vi "core_process_api_vi_ref.vi"(6 "pre/post":enum16{"pre", "post"}(ring), 8 "error in":errorcluster, 9 "vi path":path, 10 "name of caller in":string, 11 "api vi ref in":T1) -> (0 "error out":errorcluster, 3 "api vi ref out":T1)   [LabVIEW 2015]
uses:
  api_vi_ref.ctl
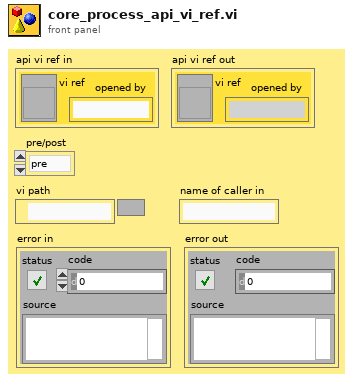
[diagram p1: front panel]
types:
  T1 = typedef "api_vi_ref.ctl" = cluster{"vi ref":refnum<vi>, "opened by":string}
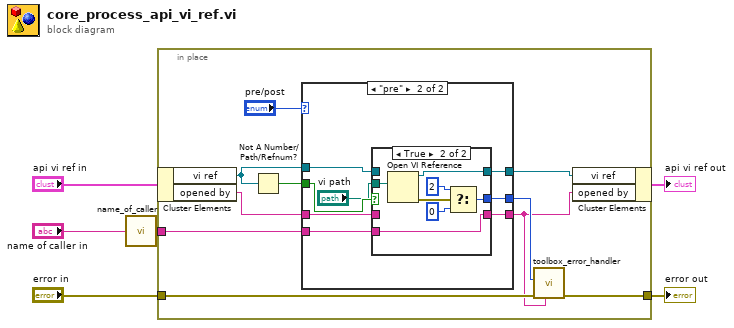
[diagram p0: block diagram]
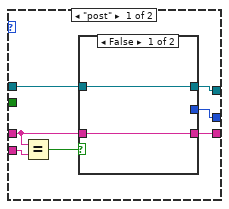
[diagram p2: hidden frame]
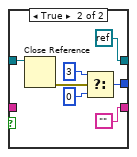
[diagram p3: hidden frame]
diagram:
  n1 = call "name_of_caller.vi"("name of caller in"="name of caller in") -> ("name of caller out"=w1:string)  [unwired: 3 in]
  n2 = in-place {
    in-place-border: [w9] -> w6
    in-place-border: "error in" -> [w10]
    in-place-border: w1 -> [w11]
    n3 = in-place-cluster #1("api vi ref in") -> ("vi ref"=w14:refnum<vi>, "opened by"=w12:string)
    n4 = Not A Number/Path/Refnum?(number/path/refnum=w14) -> (NaN/Path/Refnum?=w16:bool)
    n5 = case shown="\"pre\"" "pre/post" {
      tunnel: w16 -> [_ w38]
      tunnel: w14 -> [w23 w40]
      tunnel: [w22 w39] -> w15
      tunnel: w12 -> [w18 w34]
      tunnel: w11 -> [w21 w36]
      tunnel: [w19 w35] -> w7
      tunnel: [w17 w33] -> w8
      frame "post" {
        n6 = Equal?(x=w18, y=w21) -> (x = y?=w20:bool)
        n7 = case shown="False" w20 {
          tunnel: w23 -> [w25 w32]
          tunnel: [w25 refnum<k0> refnum] -> w22
          tunnel: [w24 ""] -> w19
          tunnel: w18 -> [w24 _]
          tunnel: [_ w26] -> w17
          frame False {
          }
          frame True {
            n8 = Close Reference(reference=w32) -> (error out=w29:errorcluster)  [unwired: 1 in]
            n9 = Select(t=3, s=w29, f=0) -> (s? t:f=w26:i32)
          }
        }
      }
      frame "pre" {
        n10 = case shown="True" w38 {
          tunnel: w40 -> [w42 _]
          tunnel: [w42 w49] -> w39
          tunnel: "vi path" -> [_ w48]
          tunnel: w36 -> [_ w47]
          tunnel: [w41 w47] -> w35
          tunnel: w34 -> [w41 _]
          tunnel: [_ w43] -> w33
          frame False {
          }
          frame True {
            n11 = Open VI Reference(vi path=w48) -> (vi reference=w49:refnum<vi>, error out=w45:errorcluster)  [unwired: 5 in]
            n12 = Select(t=2, s=w45, f=0) -> (s? t:f=w43:i32)
          }
        }
      }
    }
    n13 = call "toolbox_error_handler.vi"("name of caller in (you)"=w7, "error in (no error)"=w10, "code (0 = no error)"=w8) -> ("error out"=w9:errorcluster)  [unwired: 7 in, 1 out]
    n14 = in-place-cluster #1("vi ref"=w15, "opened by"=w7) -> (→"api vi ref out":T1)
  }
  "error out" <- w6
